vi "generate_summed_waveform.vi"(0 "Variables Cluster":T2, 1 "Cycle Count Cluster In":T5, 2 "Summed Avg Data":T6, 7 "Summed WFms In":T4, 11 "error in (no error)":errorcluster) -> (3 "Cycle Count Cluster Out":T5, 8 "Summed WFms Out":T4, 13 "Complete Data Out":T1, 15 "error out":errorcluster)   [LabVIEW 2023]
uses:
  <vilib>/Waveform/WDTOps.llb/WDT Align Waveform Timestamps DBL.vi
  <vilib>/measure/maresamp.llb/Align M + N Waveforms (single shot).vi
  <vilib>/measure/NI_MAPro.lvlib
panel:
  out "C2 Data (time)":T3
  out "C1 Data (time)":T3
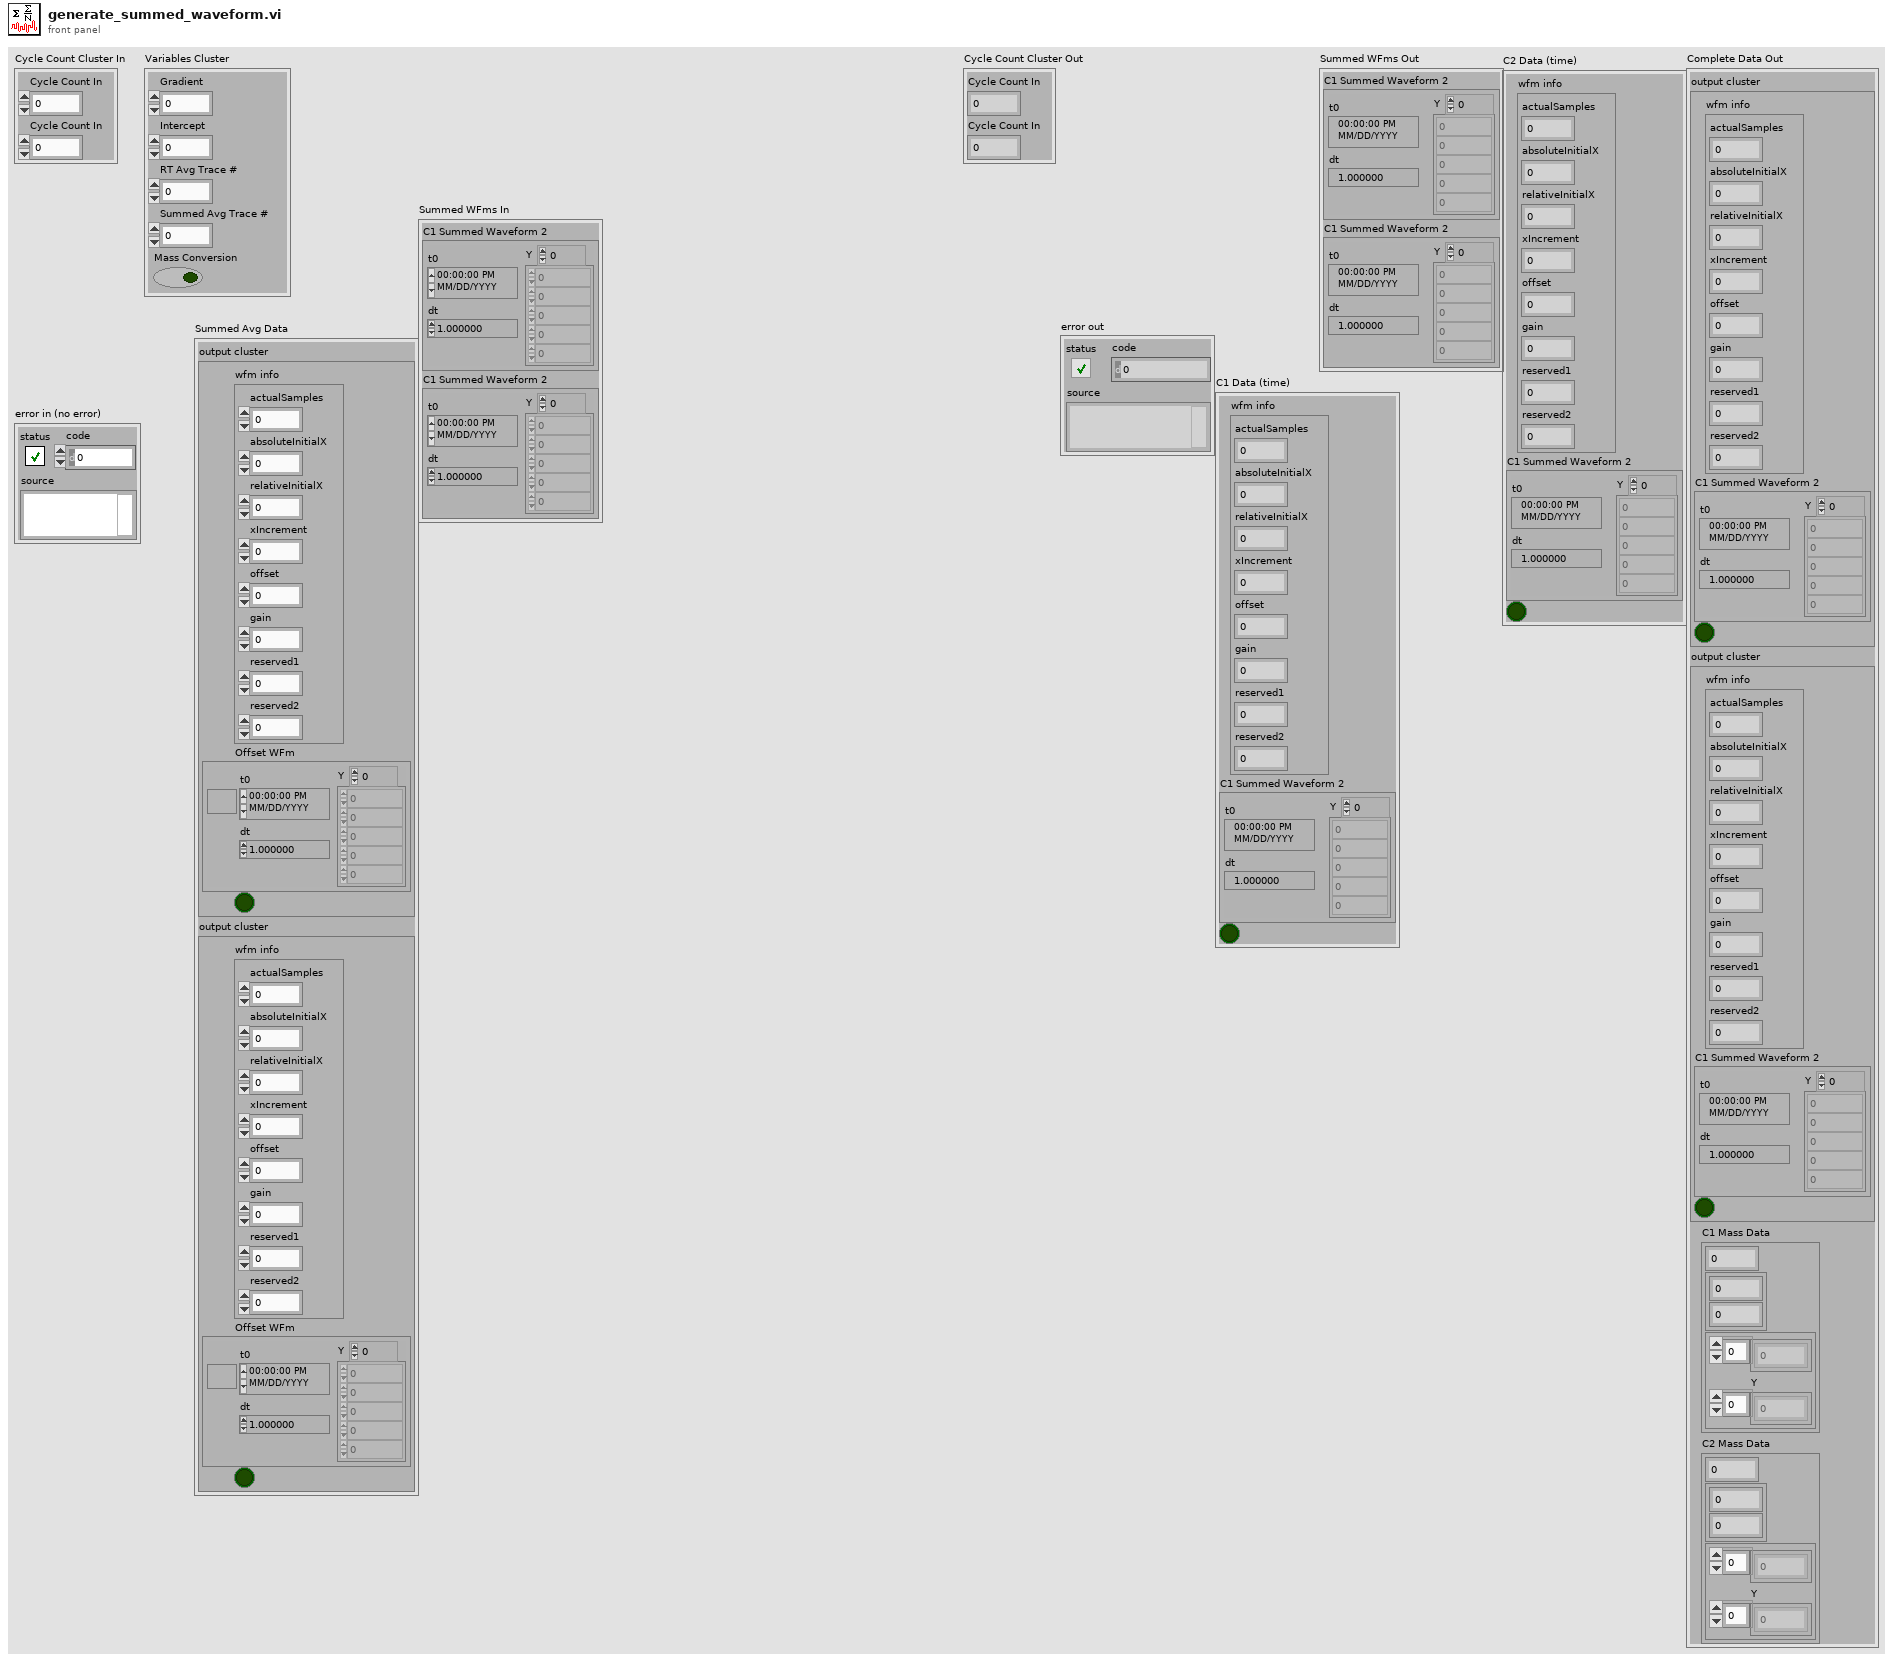
[diagram p1: front panel]
types:
  T1 = cluster{"output cluster":cluster{"wfm info":cluster{"actualSamples":i32, "absoluteInitialX":dbl, "relativeInitialX":dbl, "xIncrement":dbl, "offset":dbl, "gain":dbl, "reserved1":dbl, "reserved2":dbl}, "C1 Summed Waveform 2":waveform(dbl), bool}, "output cluster":cluster{"wfm info":cluster{"actualSamples":i32, "absoluteInitialX":dbl, "relativeInitialX":dbl, "xIncrement":dbl, "offset":dbl, "gain":dbl, "reserved1":dbl, "reserved2":dbl}, "C1 Summed Waveform 2":waveform(dbl), bool}, "C1 Mass Data":cluster{dbl, cluster{dbl, dbl}, cluster{dbl[], "Y":dbl[]}}, "C2 Mass Data":cluster{dbl, cluster{dbl, dbl}, cluster{dbl[], "Y":dbl[]}}}
  T2 = cluster{"Gradient":dbl, "Intercept":dbl, "RT Avg Trace #":i32, "Summed Avg Trace #":i32, "Mass Conversion":bool}
  T3 = cluster{"wfm info":cluster{"actualSamples":i32, "absoluteInitialX":dbl, "relativeInitialX":dbl, "xIncrement":dbl, "offset":dbl, "gain":dbl, "reserved1":dbl, "reserved2":dbl}, "C1 Summed Waveform 2":waveform(dbl), bool}
  T4 = cluster{"C1 Summed Waveform 2":waveform(dbl), "C1 Summed Waveform 2":waveform(dbl)}
  T5 = cluster{"Cycle Count In":i32, "Cycle Count In":i32}
  T6 = cluster{"output cluster":cluster{"wfm info":cluster{"actualSamples":i32, "absoluteInitialX":dbl, "relativeInitialX":dbl, "xIncrement":dbl, "offset":dbl, "gain":dbl, "reserved1":dbl, "reserved2":dbl}, "Offset WFm":waveform(dbl), bool}, "output cluster":cluster{"wfm info":cluster{"actualSamples":i32, "absoluteInitialX":dbl, "relativeInitialX":dbl, "xIncrement":dbl, "offset":dbl, "gain":dbl, "reserved1":dbl, "reserved2":dbl}, "Offset WFm":waveform(dbl), bool}}
  T7 = cluster{"wfm info":cluster{"actualSamples":i32, "absoluteInitialX":dbl, "relativeInitialX":dbl, "xIncrement":dbl, "offset":dbl, "gain":dbl, "reserved1":dbl, "reserved2":dbl}, "Offset WFm":waveform(dbl), bool}
  T8 = cluster{"actualSamples":i32, "absoluteInitialX":dbl, "relativeInitialX":dbl, "xIncrement":dbl, "offset":dbl, "gain":dbl, "reserved1":dbl, "reserved2":dbl}
  T9 = cluster{"wfm info":cluster{"actualSamples":i32, "absoluteInitialX":dbl, "relativeInitialX":dbl, "xIncrement":dbl, "offset":dbl, "gain":dbl, "reserved1":dbl, "reserved2":dbl}, waveform(dbl), bool}
  T10 = cluster{dbl, cluster{dbl, dbl}, cluster{dbl[], "Y":dbl[]}}
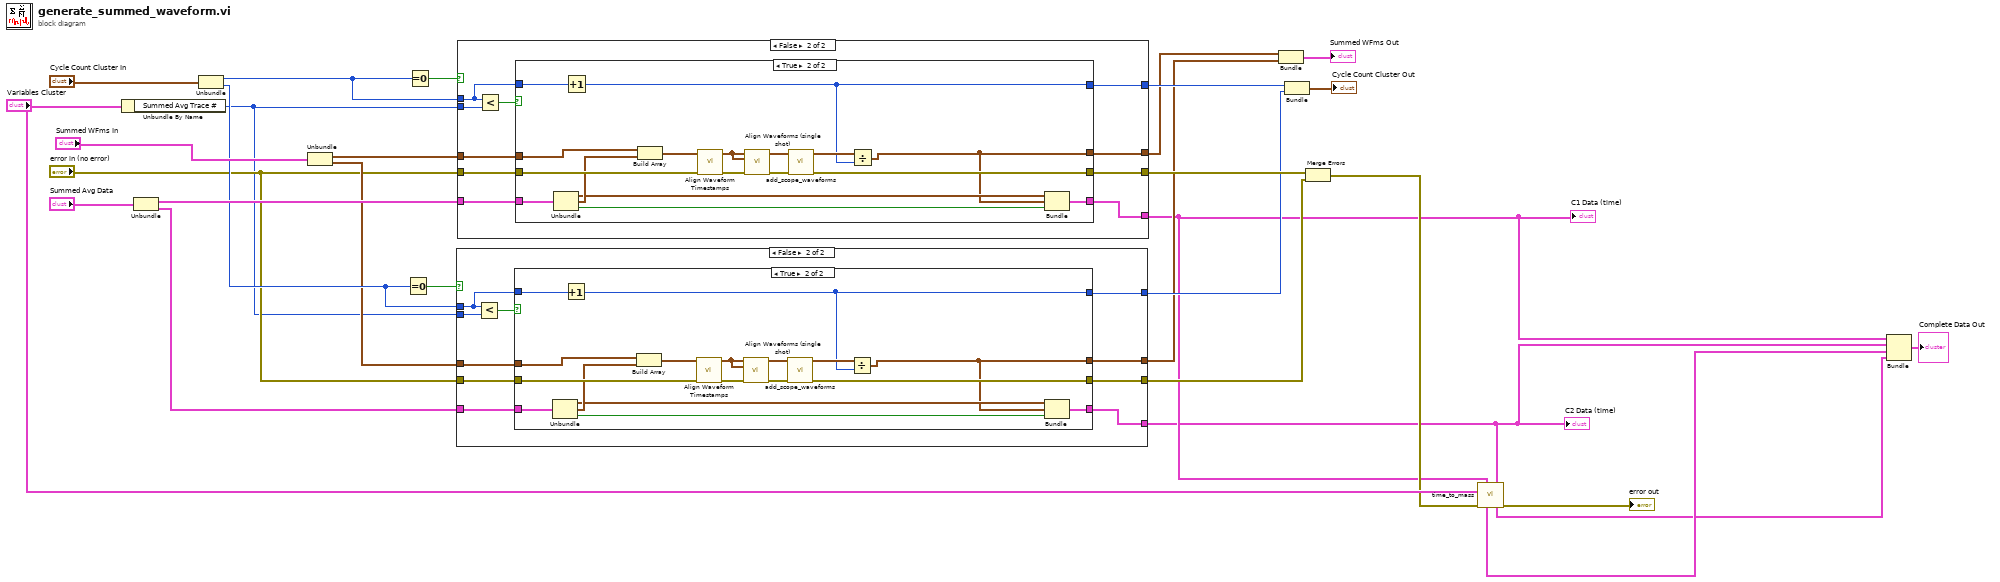
[diagram p0: block diagram]
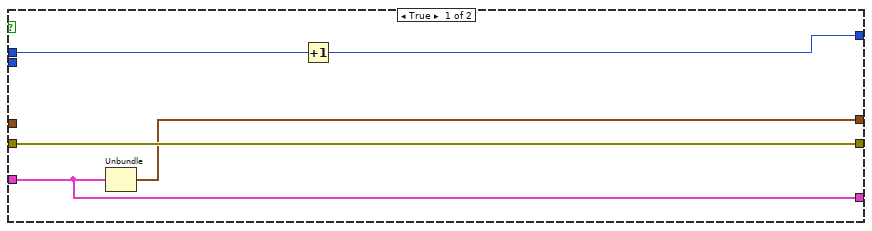
[diagram p2: hidden frame]
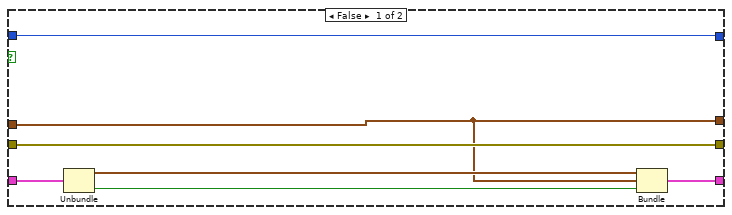
[diagram p3: hidden frame]
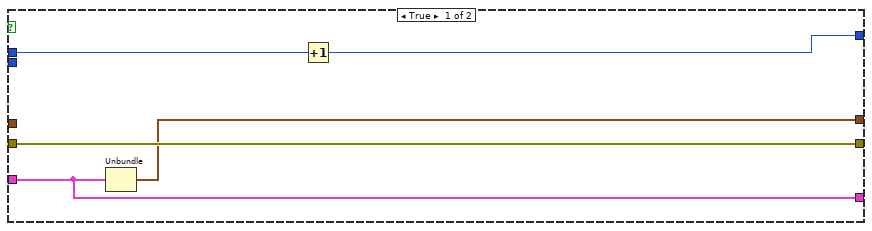
[diagram p4: hidden frame]
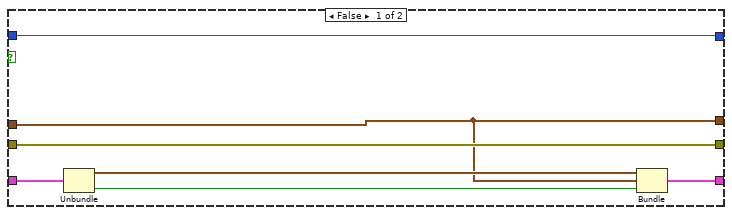
[diagram p5: hidden frame]
diagram:
  n1 = Unbundle By Name("Variables Cluster") -> ("Summed Avg Trace #"=w9:i32)
  n2 = Unbundle("Summed Avg Data") -> ("output cluster"=w26:T7, "output cluster"=w13:T7)
  n3 = Unbundle("Cycle Count Cluster In") -> ("Cycle Count In"=w24:i32, "Cycle Count In"=w16:i32)
  n4 = Unbundle("Summed WFms In") -> ("C1 Summed Waveform 2"=w20:waveform(dbl), "C1 Summed Waveform 2"=w15:waveform(dbl))
  n5 = Equal To 0?(x=w16) -> (x = 0?=w17:bool)
  n6 = Equal To 0?(x=w24) -> (x = 0?=w29:bool)
  n7 = case shown="False" w17 {
    tunnel: w16 -> [w32 w42]
    tunnel: w9 -> [_ w43]
    tunnel: [w31 w41] -> w12
    tunnel: w15 -> [_ w40]
    tunnel: w13 -> [w30 w39]
    tunnel: "error in (no error)" -> [w34 w38]
    tunnel: [w33 w37] -> w11
    tunnel: [w34 w36] -> w10
    tunnel: [w30 w35] -> w4
    frame True {
      n8 = Unbundle(w30) -> ("Offset WFm"=w33:waveform(dbl))  [unwired: 2 out]
      n9 = Increment(x=w32) -> (x+1=w31:i32)
    }
    frame False {
      n10 = Less?(x=w42, y=w43) -> (x < y?=w44:bool)
      n11 = case shown="True" w44 {
        tunnel: w42 -> [w50 w68]
        tunnel: [w50 w58] -> w41
        tunnel: w40 -> [w47 w57]
        tunnel: w39 -> [w49 w67]
        tunnel: w38 -> [w51 w65]
        tunnel: [w47 w54] -> w37
        tunnel: [w51 w60] -> w36
        tunnel: [w45 w52] -> w35
        frame False {
          n12 = Unbundle(w49) -> ("wfm info"=w48:T8, w46:bool)  [unwired: 1 out]
          n13 = Bundle("wfm info"=w48, "C1 Summed Waveform 2"=w47, w46) -> (w45:T3)  [unwired: 1 in]
        }
        frame True {
          n14 = Unbundle(w67) -> ("wfm info"=w55:T8, "Offset WFm"=w56:waveform(dbl), w53:bool)
          n15 = Increment(x=w68) -> (x+1=w58:i32)
          n16 = Build Array(w57, w56) -> (w66:waveform(dbl)[])
          n17 = call-poly <vilib>:"Align Waveform Timestamps.vi"("error in (no error)"=w65, "waveforms in"=w66) -> ("error out"=w63:errorcluster, "waveforms out"=w64:waveform(dbl)[])  [unwired: 8 in]
          n18 = call-poly <vilib>:"Align Waveforms (single shot).vi"("error in (no error)"=w63, "N waveforms in"=w64, "M waveforms in"=w64) -> ("error out"=w61:errorcluster, "M aligned waveforms out"=w62:waveform(dbl)[])  [unwired: 6 in, 1 out]
          n19 = call "add_scope_waveforms.vi"("Error in (no error)"=w61, "Waveform array"=w62) -> ("Error out"=w60:errorcluster, "Summed waveform"=w59:waveform(dbl))  [unwired: 8 in]
          n20 = Divide(x=w59, y=w58) -> (x/y=w54:waveform(dbl))
          n21 = Bundle("wfm info"=w55, w54, w53) -> (w52:T9)  [unwired: 1 in]
        }
      }
    }
  }
  "C2 Data (time)" <- w4
  n22 = case shown="False" w29 {
    tunnel: w24 -> [w71 w81]
    tunnel: w9 -> [_ w82]
    tunnel: [w70 w80] -> w23
    tunnel: w20 -> [_ w79]
    tunnel: w26 -> [w69 w78]
    tunnel: "error in (no error)" -> [w73 w77]
    tunnel: [w72 w76] -> w18
    tunnel: [w73 w75] -> w27
    tunnel: [w69 w74] -> w5
    frame True {
      n23 = Unbundle(w69) -> ("Offset WFm"=w72:waveform(dbl))  [unwired: 2 out]
      n24 = Increment(x=w71) -> (x+1=w70:i32)
    }
    frame False {
      n25 = Less?(x=w81, y=w82) -> (x < y?=w83:bool)
      n26 = case shown="True" w83 {
        tunnel: w81 -> [w89 w107]
        tunnel: [w89 w97] -> w80
        tunnel: w79 -> [w86 w96]
        tunnel: w78 -> [w88 w106]
        tunnel: w77 -> [w90 w104]
        tunnel: [w86 w93] -> w76
        tunnel: [w90 w99] -> w75
        tunnel: [w84 w91] -> w74
        frame False {
          n27 = Unbundle(w88) -> ("wfm info"=w87:T8, w85:bool)  [unwired: 1 out]
          n28 = Bundle("wfm info"=w87, "C1 Summed Waveform 2"=w86, w85) -> (w84:T3)  [unwired: 1 in]
        }
        frame True {
          n29 = Unbundle(w106) -> ("wfm info"=w94:T8, "Offset WFm"=w95:waveform(dbl), w92:bool)
          n30 = Increment(x=w107) -> (x+1=w97:i32)
          n31 = Build Array(w96, w95) -> (w105:waveform(dbl)[])
          n32 = call-poly <vilib>:"Align Waveform Timestamps.vi"("error in (no error)"=w104, "waveforms in"=w105) -> ("error out"=w102:errorcluster, "waveforms out"=w103:waveform(dbl)[])  [unwired: 8 in]
          n33 = call-poly <vilib>:"Align Waveforms (single shot).vi"("error in (no error)"=w102, "N waveforms in"=w103, "M waveforms in"=w103) -> ("error out"=w100:errorcluster, "M aligned waveforms out"=w101:waveform(dbl)[])  [unwired: 6 in, 1 out]
          n34 = call "add_scope_waveforms.vi"("Error in (no error)"=w100, "Waveform array"=w101) -> ("Error out"=w99:errorcluster, "Summed waveform"=w98:waveform(dbl))  [unwired: 8 in]
          n35 = Divide(x=w98, y=w97) -> (x/y=w93:waveform(dbl))
          n36 = Bundle("wfm info"=w94, w93, w92) -> (w91:T9)  [unwired: 1 in]
        }
      }
    }
  }
  "C1 Data (time)" <- w5
  n37 = Bundle("C1 Summed Waveform 2"=w18, "C1 Summed Waveform 2"=w11) -> (→"Summed WFms Out":T4)  [unwired: 1 in]
  n38 = Bundle("Cycle Count In"=w23, "Cycle Count In"=w12) -> (→"Cycle Count Cluster Out":T5)  [unwired: 1 in]
  n39 = Merge Errors(w27, w10) -> (w7:errorcluster)
  n40 = call "time_to_mass.vi"("C1 Data"=w5, "C2 Data"=w4, "Vairables Cluster"="Variables Cluster", "error in (no error)"=w7) -> ("C1 Mass Data"=w3:T10, "C2 Mass Data"=w2:T10, "error out"=→"error out":errorcluster)  [unwired: 9 in]
  n41 = Bundle("output cluster"=w5, "output cluster"=w4, "C1 Mass Data"=w3, "C2 Mass Data"=w2) -> (→"Complete Data Out":T1)  [unwired: 1 in]
